vi "init.vi"(8 "error in (no error)":errorcluster, 9 "ScanName":string, 10 "LogPath":path, 11 "CSVTestLog in":refnum<class "CSVTestLog.lvclass">) -> (0 "error out":errorcluster, 3 "CSVTestLog out":refnum<class "CSVTestLog.lvclass">)   [LabVIEW 2015, in "CSVTestLog.lvclass"]
uses:
  CSVTestLog.lvclass
  CSVTestLog.lvclass/CSVTestLog.ctl
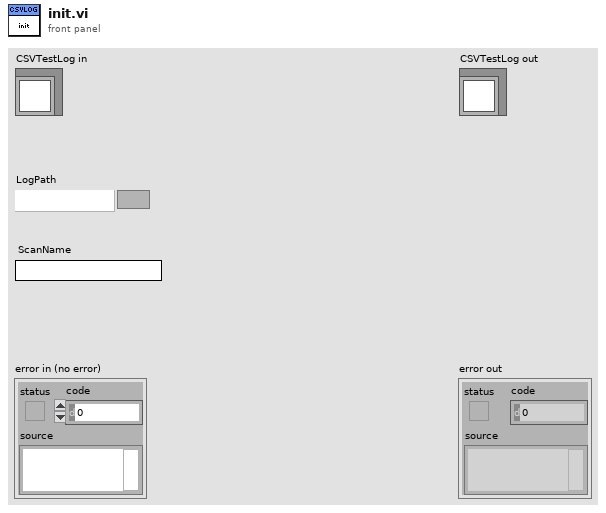
[diagram p1: front panel]
types:
  T1 = enum16{"open", "replace", "create", "open or create", "replace or create", "replace or create with confirmation"}
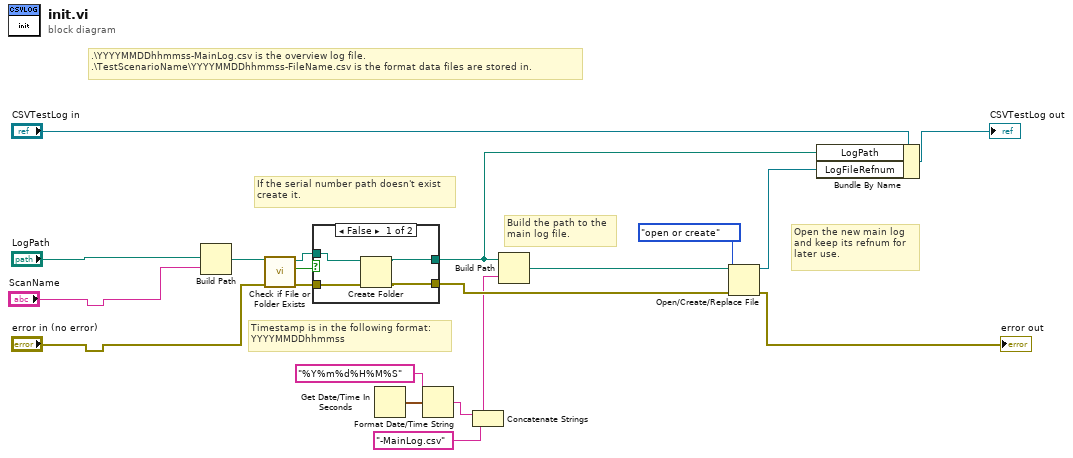
[diagram p0: block diagram]
diagram:
  # "Build the path to the\nmain log file."
  # "Open the new main log\nand keep its refnum for\nlater use."
  # "Timestamp is in the following format:\nYYYYMMDDhhmmss"
  # "If the serial number path doesn't exist\ncreate it."
  # ".\\YYYYMMDDhhmmss-MainLog.csv is the overview log file.\n.\\TestScenarioName\\YYYYMMDDhhmmss-FileName.csv is the format data files are stored in."
  n1 = Build Path(base path="LogPath", name or relative path="ScanName") -> (appended path=w15:path)
  n2 = call <vilib>:"Check if File or Folder Exists.vi"("error in (no error)"="error in (no error)", "path"=w15) -> ("error out"=w18:errorcluster, "file or folder exists?"=w16:bool, "dup path"=w17:path)  [unwired: 7 in]
  n3 = case shown="False" w16 {
    tunnel: w17 -> [w24 w26]
    tunnel: w18 -> [w23 w25]
    tunnel: [w22 w25] -> w19
    tunnel: [w21 w26] -> w20
    frame False {
      n4 = Create Folder(path (use dialog)=w24, error in=w23) -> (created path=w21:path, error out=w22:errorcluster)  [unwired: 1 in, 1 out]
    }
    frame True {
    }
  }
  n5 = Get Date/Time In Seconds() -> (seconds since 1Jan1904=w10:timestamp)
  n6 = Format Date/Time String(time format string (%c)="%Y%m%d%H%M%S", seconds (now)=w10) -> (date/time string=w12:string)  [unwired: 1 in]
  n7 = Concatenate Strings(w12, "-MainLog.csv" ("string")) -> (w8:string)
  n8 = Build Path(base path=w20, name or relative path=w8) -> (appended path=w13:path)
  n9 = Open/Create/Replace File(file path (use dialog)=w13, error in=w19, operation (0:open)=T1."open or create") -> (refnum out=w14:refnum<file>, error out=→"error out":errorcluster)  [unwired: 3 in, 1 out]
  n10 = Bundle By Name(cluster="CSVTestLog in", "LogPath"=w20, "LogFileRefnum"=w14) -> (→"CSVTestLog out":refnum<class "CSVTestLog.lvclass">)
